vi "Test Write Width.vi"() -> ()   [LabVIEW 2020, in "Rover.lvlib" / "Rover.lvclass"]
uses:
  Rover.lvclass
  I2C Register.ctl
  <vilib>/MakerHub/LINX/Private/Local IO/LinxI2cWrite.vi
  <vilib>/MakerHub/LINX/Public/Utilities/Check Channel.vi
  <vilib>/MakerHub/LINX/Private/Local IO/Handle Errors.vi
  <vilib>/MakerHub/LINX/Public/Utilities/Open Local.vi
  <vilib>/MakerHub/LINX/Private/Utilties/Generate Error.vi
  <vilib>/MakerHub/LINX/LMH-LINX.lvlib
panel:
  out "error out":errorcluster
  in  "Width in meters":sgl
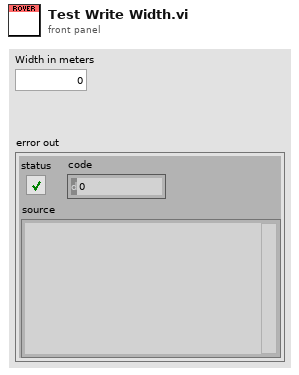
[diagram p1: front panel]
types:
  T1 = typedef "LMH-LINX.lvlib/LINX Ref.ctl" = cluster{"IO":T2, "Interface":T3, "LINX Device Config":T4}
  T2 = typedef "LMH-LINX.lvlib/Platform.ctl" = enum16{"Remote", "Local"}
  T3 = typedef "LMH-LINX.lvlib/Interface.ctl" = enum16{"Serial", "TCP"}
  T4 = typedef "LMH-LINX.lvlib/Device.lvlib/LINX Device Config.ctl" = cluster{"Interface":T3, "COM Port":refnum<visa-resource-name>, "TCP Configuration":T5, "Device Family":u8, "Device ID":u8, "Device Name":string, "TCP Ref":refnum<k5>, "Channels":T6}
  T5 = typedef "LMH-LINX.lvlib/Device.lvlib/TCP Config.ctl" = cluster{"IP Address":string, "Port":u16}
  T6 = typedef "LMH-LINX.lvlib/Channels.ctl" = cluster{"DI":u8[], "DO":u8[], "AI":u8[], "AO":u8[], "PWM":u8[], "QE":u8[], "UART":u8[], "I2C 2":u8[], "SPI":u8[], "CAN":u8[], "Servo":u8[], "AI Ref (V)":dbl, "AI Resolution (Bits)":u8, "AO Ref (V)":dbl, "AO Resolution (Bits)":u8}
  T7 = typedef "Rover.lvlib/Rover.lvclass/I2C Register.ctl" = enum8{"encA", "encB", "ticksPerUnit", "width", "flags", "velP", "velI", "velD", "velMin", "velMax", "poseX", "poseY", "poseA", "cmdDrive", "cmdTurn", "velocity", "turn", "velL", "velR", "run", "outL", "outR", "outDeadband"}
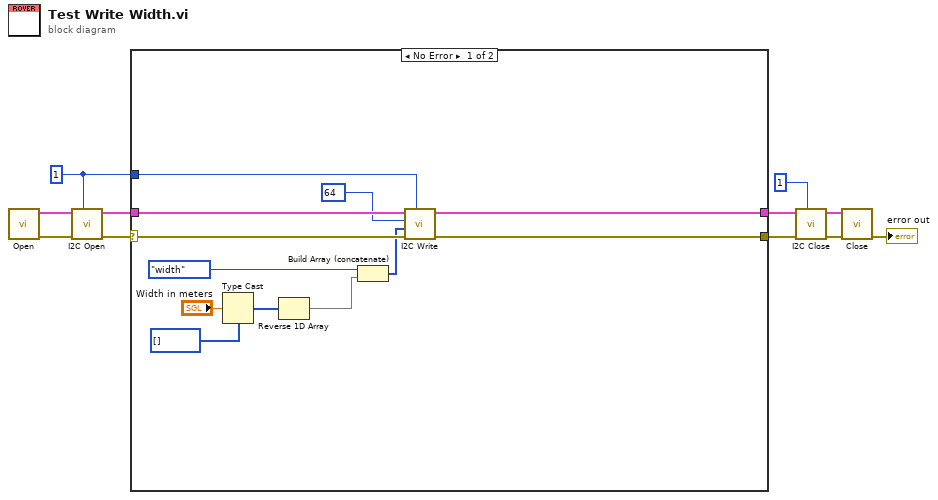
[diagram p0: block diagram]
diagram:
  w2 = u8 1 ("I2C Channel (0)")
  n1 = call-poly <vilib>:"Open.vi"() -> ("Error Out"=w10:errorcluster, "LINX Resource"=w11:T1)  [unwired: 9 in, 1 out]
  n2 = call <vilib>:"I2C Open.vi"("I2C Channel (0)"=w2, "Error In"=w10, "LINX Resource"=w11) -> ("Error Out"=w9:errorcluster, "LINX Resource"=w8:T1)  [unwired: 7 in]
  n3 = case shown="No Error" w9 {
    selector: w9 -> [w22 w25]
    tunnel: w8 -> [w23 w24]
    tunnel: [w14 w25] -> w6
    tunnel: [w15 w24] -> w7
    tunnel: w2 -> [w16 _]
    frame No Error {
      n4 = Type Cast(type=u8[] [], x="Width in meters") -> (*(type *) &x=w13:u8[])
      n5 = Reverse 1D Array(array=w13) -> (reversed array=w12:u8[])
      n6 = Build Array (concatenate)(I2C_Register."width" ("I2C Register"), w12) -> (w18:u8[])
      n7 = call <vilib>:"I2C Write.vi"("I2C Channel"=w16, "Error In"=w22, "Data"=w18, "I2C Slave Address (0)"=u8 64, "LINX Resource"=w23) -> ("Error Out"=w14:errorcluster, "LINX Resource"=w15:T1)  [unwired: 5 in]
    }
    frame Error {
    }
  }
  n8 = call <vilib>:"I2C Close.vi"("I2C Channel (0)"=u8 1, "Error In"=w6, "LINX Resource"=w7) -> ("Error Out"=w3:errorcluster, "LINX Resource"=w4:T1)  [unwired: 7 in]
  n9 = call <vilib>:"Close.vi"("Error In"=w3, "LINX Resource"=w4) -> ("Error Out"=→"error out":errorcluster)  [unwired: 9 in]
